vi "photo_encoder_new3.vi"() -> ()   [LabVIEW 2014]
panel:
  out "i+100":dbl
  out "i":dbl
  out "Marks/second":dbl
  in  "Brightness of Mark":dbl
  in  "Photo Value(placeholder for sensor data)":dbl
  # "This VI recognizes significant increases in brightness as \"marks\" and outputs the number of marks detected in the last second.\nKnown issue:  Workaround failed, so i+100 is always i, and marks/second is decremented when it shouldn't be.  Now that I think about it, further tweaking of the workaround probably won't yield results."
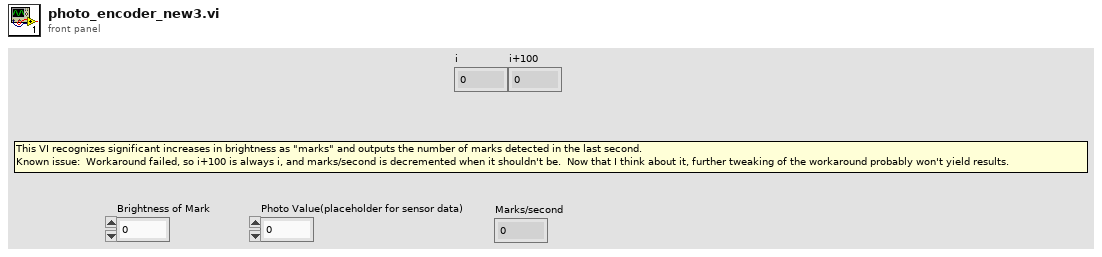
[diagram p1: front panel]
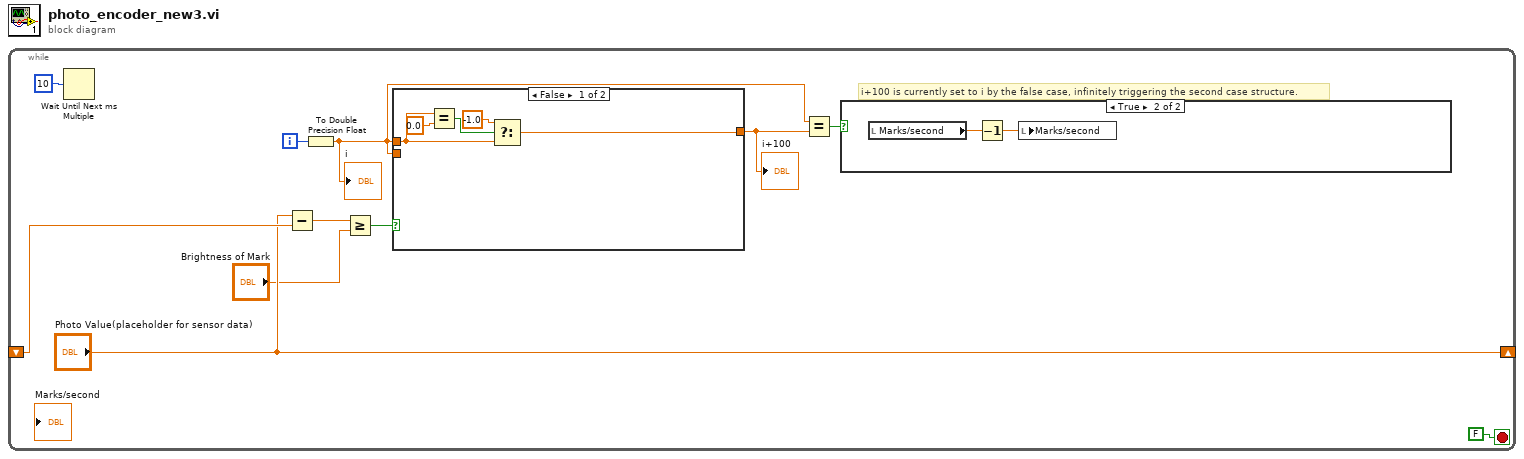
[diagram p0: block diagram]
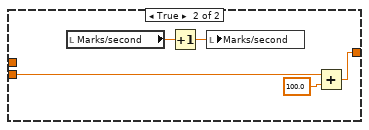
[diagram p3: hidden frame]
diagram:
  n1 = while {
    shift-right: ["Photo Value(placeholder for sensor data)"] -> _
    shift-left: _ -> [w11]
    i -> [w2]
    stop <- FALSE stop-if-true
    # "i+100 is currently set to i by the false case, infinitely triggering the second case structure."
    n2 = Wait Until Next ms Multiple(millisecond multiple=u32 10) -> ()  [unwired: 1 out]
    n3 = Subtract(x="Photo Value(placeholder for sensor data)", y=w11) -> (x-y=w9:dbl)
    n4 = To Double Precision Float(number=w2) -> (double precision float=w1:dbl)
    "i" <- w1
    n5 = Greater Or Equal?(x=w9, y="Brightness of Mark") -> (x >= y?=w7:bool)
    n6 = case shown="False" w7 {
      tunnel: [w16 w21] -> w3
      tunnel: w1 -> [_ w20]
      tunnel: w1 -> [w14 _]
      frame False {
        n7 = Equal?(x=w14, y=0.0) -> (x = y?=w17:bool)
        n8 = Select(t=-1.0, s=w17, f=w14) -> (s? t:f=w16:dbl)
      }
      frame True {
        n9 = local read "Marks/second"() -> (w22:dbl)
        n10 = Increment(x=w22) -> (x+1=w23:dbl)
        n11 = local write "Marks/second"(w23) -> ()
        n12 = Add(x=w20, y=100.0) -> (x+y=w21:dbl)
      }
    }
    "i+100" <- w3
    n13 = Equal?(x=w1, y=w3) -> (x = y?=w4:bool)
    n14 = case shown="True" w4 {
      frame False {
      }
      frame True {
        n15 = local read "Marks/second"() -> (w12:dbl)
        n16 = Decrement(x=w12) -> (x-1=w13:dbl)
        n17 = local write "Marks/second"(w13) -> ()
      }
    }
  }
